vi "Read (Multiple Points).vi"(0 "VISA resource name":refnum<visa-resource-name>, 5 "Maximum Time (30000 ms)":u32=30000, 7 "Sample Count (1)":i32=1 format="%#.6g", 9 "Trigger Count (1)":i32=1 format="%#.6g", 11 "error in (no error)":errorcluster) -> (4 "VISA resource name out":refnum<visa-resource-name>, 6 "Measurements":dbl[](array[numeric]), 15 "error out":errorcluster)   [LabVIEW 2022 SP3, in "Agilent 34420.lvlib"]
doc: "Reads and returns multiple measurements from the instrument. Use this VI when you want to take multiple measurements. Use the low-level VIs for other triggering options."
uses:
  Agilent 34420.lvlib
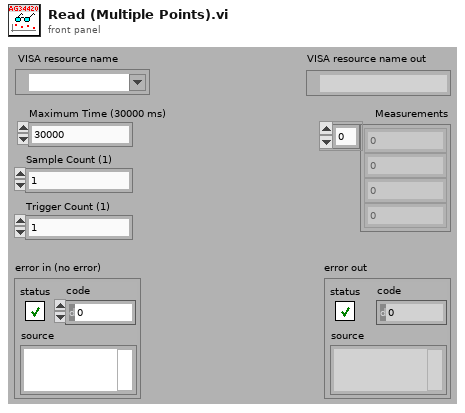
[diagram p1: front panel]
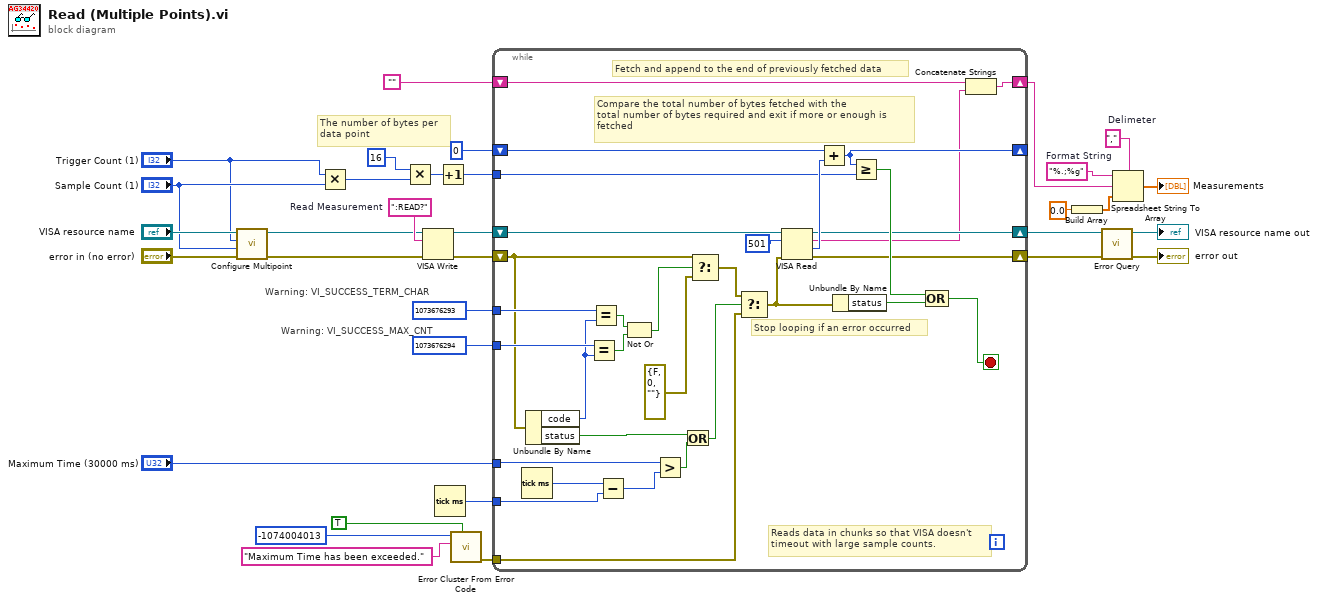
[diagram p0: block diagram]
diagram:
  w30 = ","  # Delimeter
  w31 = "%.;%g"  # Format String
  w26 = ":READ?"  # Read Measurement
  # "The number of bytes per\ndata point"
  # "Warning: VI_SUCCESS_MAX_CNT"
  # "Warning: VI_SUCCESS_TERM_CHAR"
  n1 = call "Configure Multipoint.vi"("error in (no error)"="error in (no error)", "Sample Count (1)"="Sample Count (1)", "Trigger Count (1)"="Trigger Count (1)", "VISA resource name"="VISA resource name") -> ("error out"=w1:errorcluster, "VISA resource name out"=w2:refnum<visa-resource-name>)  [unwired: 6 in]
  n2 = Multiply(x="Trigger Count (1)", y="Sample Count (1)") -> (x*y=w3:i32)
  n3 = Multiply(x=16, y=w3) -> (x*y=w9:i32)
  n4 = VISA Write(VISA resource name=w2, write buffer=w26, error in (no error)=w1) -> (VISA resource name out=w13:refnum<visa-resource-name>, error out=w14:errorcluster)  [unwired: 1 out]
  n5 = Tick Count (ms)() -> (millisecond timer value=w21:u32)
  n6 = Increment(x=w9) -> (x+1=w8:i32)
  n7 = call <vilib>:"Error Cluster From Error Code.vi"("show call chain? (False)"=TRUE, "error message (\"\")"="Maximum Time has been exceeded." ("error message (\"\")"), "error code (0)"=-1074004013) -> ("error out"=w20:errorcluster)  [unwired: 6 in]
  n8 = while {
    shift-right: [w41] -> w11
    shift-left: w13 -> [w47]
    shift-right: [w42] -> w12
    shift-left: w14 -> [w62]
    tunnel: w8 -> [w38]
    tunnel: 1073676293 -> [w64]
    tunnel: 1073676294 -> [w63]
    tunnel: w21 -> [w56]
    tunnel: "Maximum Time (30000 ms)" -> [w54]
    tunnel: w20 -> [w50]
    shift-right: [w40] -> _
    shift-left: 0 -> [w39]
    shift-right: [w36] -> w15
    shift-left: "" -> [w35]
    stop <- w48 stop-if-true
    # "Stop looping if an error occurred"
    # "Reads data in chunks so that VISA doesn't\ntimeout with large sample counts."
    # "Compare the total number of bytes fetched with the \ntotal number of bytes required and exit if more or enough is\nfetched"
    # "Fetch and append to the end of previously fetched data"
    n9 = Tick Count (ms)() -> (millisecond timer value=w57:u32)
    n10 = Unbundle By Name(w62) -> ("code"=w61:i32, "status"=w53:bool)
    n11 = Equal?(x=w63, y=w61) -> (x = y?=w59:bool)
    n12 = Equal?(x=w64, y=w61) -> (x = y?=w60:bool)
    n13 = Subtract(x=w57, y=w56) -> (x-y=w55:u32)
    n14 = Not Or(1:w59, 2:w60) -> (0:w58:bool)
    n15 = Greater?(x=w54, y=w55) -> (0:w52:bool)
    n16 = Or(x=w53, y=w52) -> (x .or. y?=w51:bool)
    n17 = Select(t=w62, s=w58, f=errorcluster {"status"=FALSE, "code"=0, "source"=""}) -> (s? t:f=w46:errorcluster)
    n18 = Select(t=w46, s=w51, f=w50) -> (s? t:f=w37:errorcluster)
    n19 = VISA Read(VISA resource name=w47, byte count=u32 501, error in (no error)=w37) -> (VISA resource name out=w41:refnum<visa-resource-name>, read buffer=w34:string, return count=w44:u32, error out=w42:errorcluster)
    n20 = Add(x=w39, y=w44) -> (x+y=w40:u32)
    n21 = Unbundle By Name(w37) -> ("status"=w49:bool)
    n22 = Greater Or Equal?(x=w40, y=w38) -> (x >= y?=w43:bool)
    n23 = Compound Arithmetic op=OR(w43, w49) -> (w48:bool)
    n24 = Concatenate Strings(w35, w34) -> (w36:string)
  }
  n25 = Build Array(0.0) -> (w28:dbl[])
  n26 = call "Error Query.vi"("error in (no error)"=w12, "VISA resource name"=w11) -> ("error out"=→"error out":errorcluster, "VISA resource name out"=→"VISA resource name out":refnum<visa-resource-name>)  [unwired: 6 in, 2 out]
  n27 = Spreadsheet String To Array(delimiter (Tab)=w30, format string=w31, spreadsheet string=w15, array type (2D Dbl)=w28) -> (array=→"Measurements":dbl[])
